vi "Read Connection Configuration.vi"(8 "error in (no error)":errorcluster, 11 "SystemLink configuration in":refnum<class "SystemLink File configuration.lvclass">) -> (0 "error out":errorcluster, 2 "Connection Configuration":T1, 3 "SystemLink configuration out":refnum<class "SystemLink File configuration.lvclass">)   [LabVIEW 2015, in "SystemLink File configuration.lvclass"]
uses:
  SystemLink File configuration.lvclass
  Connection Configuration.ctl
  Connection Type.ctl
  SystemLink File configuration.lvclass/SystemLink File configuration.ctl
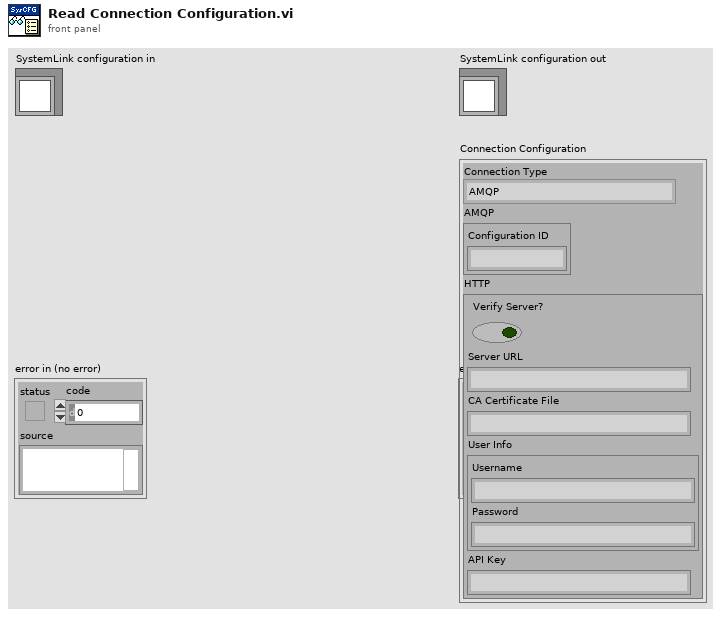
[diagram p1: front panel]
types:
  T1 = typedef "SystemLink File configuration.lvclass/Connection Configuration.ctl" = cluster{"Connection Type":T2, "AMQP":cluster{"Configuration ID":string}, "HTTP":cluster{"Verify Server?":bool, "Server URL":string, "CA Certificate File":string, "User Info":cluster{"Username":string, "Password":string}, "API Key":string}}
  T2 = typedef "SystemLink File configuration.lvclass/Connection Type.ctl" = enum16{"AMQP", "HTTP", "API Key (SystemLink Cloud)"}
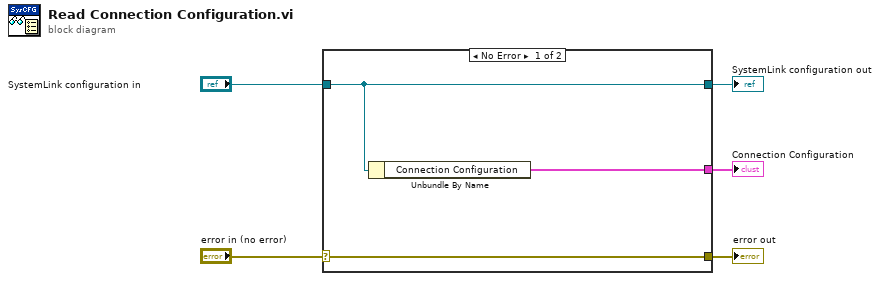
[diagram p0: block diagram]
diagram:
  n1 = case shown="No Error" "error in (no error)" {
    selector: "error in (no error)" -> [w8 w9]
    tunnel: [w8 w9] -> w4
    tunnel: [w7 w10] -> w2
    tunnel: "SystemLink configuration in" -> [w7 w10]
    tunnel: [w6 _] -> w1
    frame No Error {
      n2 = Unbundle By Name(w7) -> ("Connection Configuration"=w6:T1)
    }
    frame Error {
    }
  }
  "error out" <- w4
  "SystemLink configuration out" <- w2
  "Connection Configuration" <- w1
